vi "ADAM_Server_Channels.vi"() -> ()   [LabVIEW 2014]
uses:
  ADAM Client/Sub VIs/ADAM Controls/Search_mode.ctl
  <vilib>/Analysis/baseanly.llb/Mean (DBL).vi
  Globals/Meas_global.vi
  <vilib>/Analysis/NI_AALBase.lvlib
panel:
  out "Waveform Graph":dbl[][](graph)
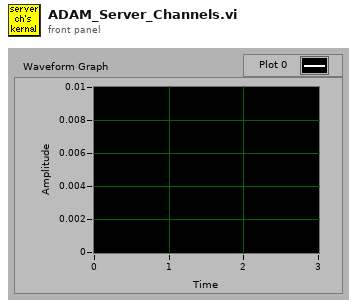
[diagram p1: front panel]
types:
  T1 = typedef "Analysis_info_cluster.ctl" = cluster{"Colour":u32, "Inst type":T2, "Inst name":string, "Symbol":string, "Code name":string, "Extra Info":string, "Inst Array":T3, "Extra Titles":string[], "Extra Values":string[], "U":dbl, "u^2":dbl, "u^3":dbl, "u^4":dbl, "Skew_u":dbl, "Kurt_u":dbl, "Sd Error in Mean":dbl, "% u'/U":dbl, "X":dbl, "Y":dbl, "Z":dbl, "Timescale integral to 25%":dbl, "Sd Error in Variance":dbl, "Calib File":path, "Calib Constants":dbl[], "Output Position":bool, "Full Stats":bool, "Av Sampling Rate":dbl, "Av No of Samples":dbl, "Total Meas Time (s)":dbl, "ADAM Ch Name":string}
  T2 = typedef "Inst_type.ctl" = enum16{"Propeller anemometer", "Raw voltage", "Pressure Transducer", "Pitot-static tube", "Preston tube", "Hot wire", "Cross wire 1", "Cross wire 2", "Generic Linear", "Generic Polynomial", "Generic BackPoly", "Fast FID", "Thermocouple", "Cold wire", "Pulsed Wire", "LDA Vel", "LDA Tran time", "LDA Arr time"}
  T3 = typedef "Instrument_Array.ctl" = enum16{"PWA", "LDA", "Analogue"}
  T4 = typedef "Search_mode.ctl" = enum16{"Between times", "All Times"}
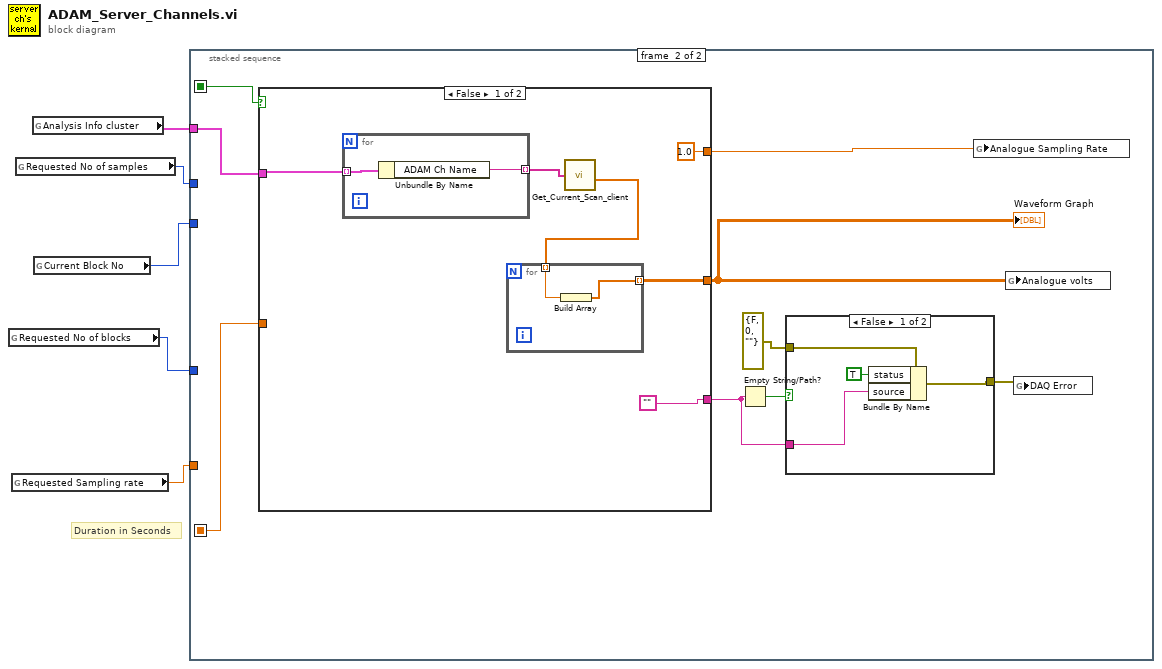
[diagram p0: block diagram]
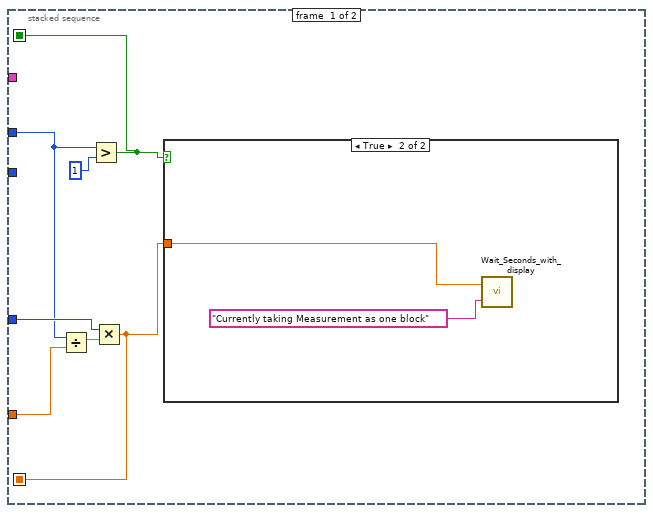
[diagram p2: hidden frame]
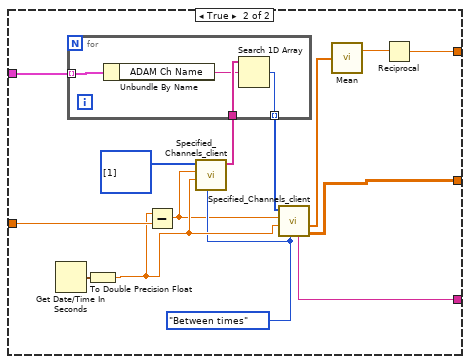
[diagram p4: hidden frame]
diagram:
  # "Duration in Seconds"
  n1 = global read "Meas_global.vi" "Requested No of blocks"() -> (w1:i32)
  n2 = global read "Meas_global.vi" "Requested Sampling rate"() -> (w4:dbl)
  n3 = global read "Meas_global.vi" "Requested No of samples"() -> (w5:i32)
  n4 = global read "Meas_global.vi" "Analysis Info cluster"() -> (w2:T1[])
  n5 = global read "Meas_global.vi" "Current Block No"() -> (w3:i32)
  n6 = stacked-sequence {
    seq-local: [w9 _] -> [_ w23]
    seq-local: [w6 _] -> [_ w15]
    tunnel: w5 -> [w8 _]
    tunnel: w3 -> [_ _]
    tunnel: w2 -> [_ w21]
    tunnel: w4 -> [w12 _]
    tunnel: w1 -> [w10 _]
    frame #0 {
      n7 = Divide(x=w8, y=w12) -> (x/y=w11:dbl)
      n8 = Greater?(x=w8, y=1) -> (0:w6:bool)
      n9 = Multiply(x=w10, y=w11) -> (x*y=w9:dbl)
      n10 = case shown="True" w6 {
        tunnel: w9 -> [_ w13]
        frame False {
        }
        frame True {
          n11 = call "Wait_Seconds_with_display.vi"("Message"="Currently taking Measurement as one block", "Seconds to wait"=w13) -> ()  [unwired: 2 out]
        }
      }
    }
    frame #1 {
      n12 = case shown="False" w15 {
        tunnel: w23 -> [_ w46]
        tunnel: [w26 w39] -> w22
        tunnel: w21 -> [w29 w38]
        tunnel: [1.0 w35] -> w20
        tunnel: ["" w34] -> w16
        frame False {
          n13 = for {
            tunnel: w29 -> [w33] mode=indexing
            tunnel: [w32] -> w28 mode=indexing
            n14 = Unbundle By Name(w33) -> ("ADAM Ch Name"=w32:string)
          }
          n15 = call "Get_Current_Scan_client.vi"("ADAM Ch Names"=w28) -> ("Numerical Values"=w27:dbl[])  [unwired: 1 in, 2 out]
          n16 = for {
            tunnel: w27 -> [w31] mode=indexing
            tunnel: [w30] -> w26 mode=indexing
            n17 = Build Array(w31) -> (w30:dbl[])
          }
        }
        frame True {
          w41 = Search_mode."Between times" ("Mode")
          n18 = Get Date/Time In Seconds() -> (seconds since 1Jan1904=w47:timestamp)
          n19 = To Double Precision Float(number=w47) -> (double precision float=w45:dbl)
          n20 = Subtract(x=w45, y=w46) -> (x-y=w40:dbl)
          n21 = call "Specified_Channels_client.vi"("Mode"=w41, "End time"=w45, "Start time"=w40, "ADAM Index array"=i32[] [1]) -> ("All Active Ch Names"=w43:string[])  [unwired: 1 in, 6 out]
          n22 = for {
            tunnel: w38 -> [w51] mode=indexing
            tunnel: w43 -> [w50]
            tunnel: [w48] -> w42 mode=indexing
            n23 = Unbundle By Name(w51) -> ("ADAM Ch Name"=w49:string)
            n24 = Search 1D Array(1D array=w50, element=w49) -> (index of element=w48:i32)  [unwired: 1 out]
          }
          n25 = call "Specified_Channels_client.vi"("Mode"=w41, "End time"=w45, "Start time"=w40, "ADAM Index array"=w42) -> ("Output array"=w39:dbl[][], "Averaging Period"=w37:dbl[], "Messages"=w34:string)  [unwired: 1 in, 4 out]
          n26 = call-poly <vilib>:"Mean.vi"("X"=w37) -> ("mean"=w36:dbl)  [unwired: 1 out]
          n27 = Reciprocal(x=w36) -> (1/x=w35:dbl)
        }
      }
      "Waveform Graph" <- w22
      n28 = Empty String/Path?(string/path=w16) -> (empty?=w19:bool)
      n29 = case shown="False" w19 {
        tunnel: errorcluster {"status"=FALSE, "code"=0, "source"=""} ("DAQ Error") -> [w55 w56]
        tunnel: [w54 w56] -> w17
        tunnel: w16 -> [w52 _]
        frame False {
          n30 = Bundle By Name(cluster=w55, "status"=TRUE, "source"=w52) -> (w54:errorcluster)
        }
        frame True {
        }
      }
      n31 = global write "Meas_global.vi" "Analogue Sampling Rate"(w20) -> ()
      n32 = global write "Meas_global.vi" "Analogue volts"(w22) -> ()
      n33 = global write "Meas_global.vi" "DAQ Error"(w17) -> ()
    }
  }
